vi "Vider et enregistrer datas.vi"(8 "error in (no error)":errorcluster caption="entrée d'erreur (pas d'erreur)", 11 "Maestro Data Logg en entrée":refnum<class "Maestro Data Logg.lvclass">) -> (0 "error out":errorcluster caption="sortie d'erreur", 3 "Maestro Data Logg en sortie":refnum<class "Maestro Data Logg.lvclass">)   [LabVIEW 2021, in "Maestro Data Logg.lvclass"]
uses:
  Maestro Data Logg.lvclass
  Maestro Data Logg.lvclass/Maestro Data Logg.ctl
panel:
  out "nb d'éléments dans la file d'attente":i32
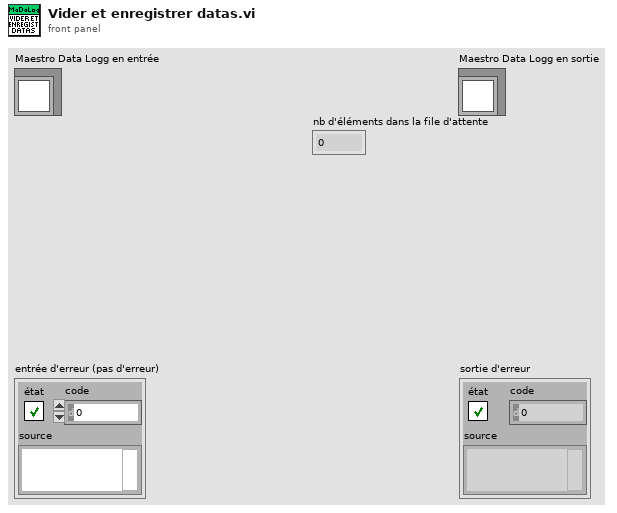
[diagram p1: front panel]
types:
  T1 = cluster{"Tps(s)":dbl[], "Puiss.":dbl, "Waveform":waveform(dbl)[], "Temps H:M:S":string[]}[]
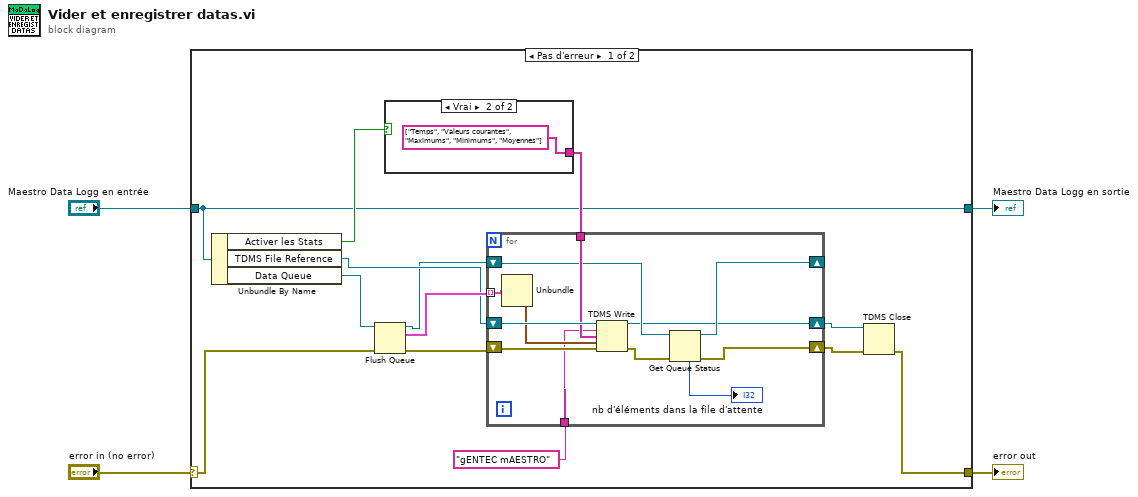
[diagram p0: block diagram]
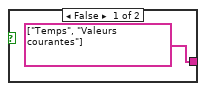
[diagram p2: hidden frame]
diagram:
  n1 = case shown="Pas d'erreur" "error in (no error)" {
    selector: "error in (no error)" -> [w10 w33]
    tunnel: [w7 w33] -> w3
    tunnel: [w9 w32] -> w1
    tunnel: "Maestro Data Logg en entrée" -> [w9 w32]
    frame No Error {
      n2 = Unbundle By Name(w9) -> ("Activer les Stats"=w11:bool, "TDMS File Reference"=w14:refnum<k34>, "Data Queue"=w13:refnum<queue>)
      n3 = Flush Queue(queue=w13, error in (no error)=w10) -> (queue out=w8:refnum<queue>, remaining elements=w17:T1, error out=w15:errorcluster)
      n4 = case shown="Vrai" w11 {
        tunnel: [string[] ["Temps", "Valeurs courantes"] ("nom des voies en entrée (Sans titre)") string[] ["Temps", "Valeurs courantes", "Maximums", "Minimums", "Moyennes"] ("nom des voies en entrée (Sans titre)")] -> w12
        frame False {
        }
        frame True {
        }
      }
      n5 = for {
        shift-right: [w21] -> w6
        shift-left: w15 -> [w31]
        shift-right: [w20] -> w5
        shift-left: w14 -> [w30]
        tunnel: w17 -> [w29] mode=indexing
        tunnel: w12 -> [w27]
        tunnel: "gENTEC mAESTRO" ("nom du groupe en entrée (Sans titre)") -> [w26]
        shift-right: [w23] -> _
        shift-left: w8 -> [w24]
        n6 = Unbundle(w29) -> ("Waveform"=w28:waveform(dbl)[])  [unwired: 3 out]
        n7 = TDMS Write(0:w30, 5:w26, 7:w27, 9:w28, 11:w31) -> (4:w20:refnum<k34>, 15:w25:errorcluster)  [unwired: 1 in, 2 out]
        n8 = Get Queue Status(queue=w24, error in (no error)=w25) -> (queue out=w23:refnum<queue>, error out=w21:errorcluster, # elements in queue=→"nb d'éléments dans la file d'attente":i32)  [unwired: 1 in, 5 out]
      }
      n9 = TDMS Close(8:w6, 11:w5) -> (0:w7:errorcluster)  [unwired: 1 out]
    }
    frame Error {
    }
  }
  "error out" <- w3
  "Maestro Data Logg en sortie" <- w1
